vi "MALT132 output counter.vi"() -> ()   [LabVIEW 2018]
uses:
  <instrlib>/AltonTech MALT/Public/Types/MALT Family Codes.ctl
  <instrlib>/AltonTech MALT/AltonTech MALT200817.lvlib
panel:
  in  "Save":bool
  out "Kn Counter":u32
  in  "Address":i32=3 format="%02x"
  in  "Kn":i32=1
  in  "Kn":bool
  in  "stop":bool
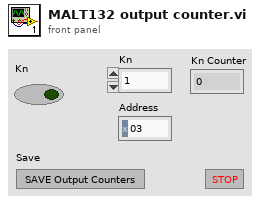
[diagram p1: front panel]
types:
  T1 = typedef "AltonTech MALT200817.lvlib/MALT Family Codes.ctl" = enum32{"-", "MALT40IO", "YAV904X8", "MALT132", "YAV91616", "MALT16PIN", "YAV90096", "YAV90HVT", "YAV90CLR", "YAV90128", "YAV90PNE", "MALTCON", "YAV91775", "YAV90XXX", "YAV90MMU", "H730050", "H710060", "H710061", "YAV90304", "MMI", "YAV90060", "MALT160T", "YAV90059", "Not Defined"}
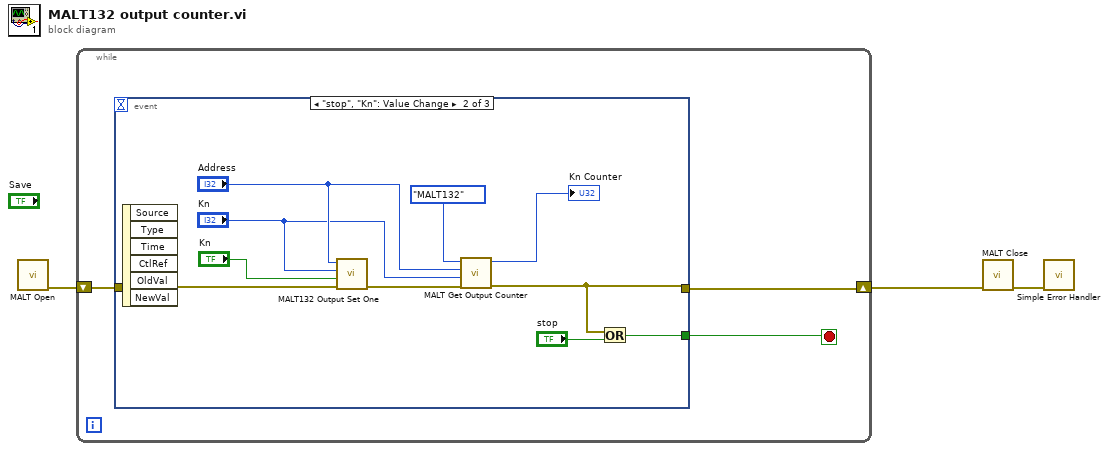
[diagram p0: block diagram]
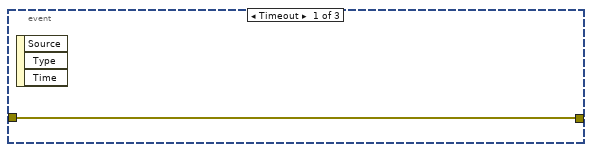
[diagram p2: hidden frame]
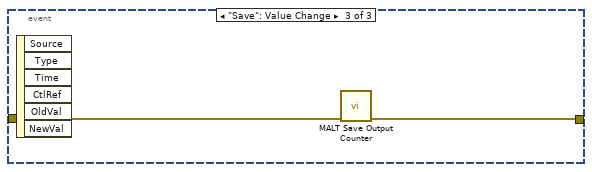
[diagram p3: hidden frame]
diagram:
  n1 = call <instrlib>:"MALT Open.vi"() -> ("error out"=w3:errorcluster)  [unwired: 10 in, 1 out]
  n2 = while {
    shift-right: [w5] -> w2
    shift-left: w3 -> [w6]
    stop <- w4 stop-if-true
    n3 = event shown="[1] \"stop\", \"Kn\": Value Change" {
      selector: _ -> [_ _ _]
      dyn-events: _ -> [_ _ _]
      timeout: _ -> [_ _ _]
      tunnel: w6 -> [w7 w16 w19]
      tunnel: [w7 w11 w18] -> w5
      tunnel: [_ w8 _] -> w4
      event Timeout {
        n4 = event-data() -> ()  [unwired: 1 in, 3 out]
      }
      event "stop", "Kn": Value Change {
        n5 = event-data() -> ()  [unwired: 1 in, 6 out]
        n6 = call <instrlib>:"MALT132 Output Set One.vi"("error in"=w16, "State"="Kn", "Kn"="Kn", "Address"="Address") -> ("error out"=w15:errorcluster)  [unwired: 7 in]
        n7 = call <instrlib>:"MALT Get Output Counter.vi"("error in"=w15, "Port"="Kn", "Address"="Address", "FamilyCode"=MALT_Family_Codes."MALT132") -> ("error out"=w11:errorcluster, "Value"=→"Kn Counter":u32)  [unwired: 6 in]
        n8 = Or(x=w11, y="stop") -> (x .or. y?=w8:bool)
      }
      event "Save": Value Change {
        n9 = event-data() -> ()  [unwired: 1 in, 6 out]
        n10 = call <instrlib>:"MALT Save Output Counter.vi"("error in"=w19) -> ("error out"=w18:errorcluster)  [unwired: 10 in]
      }
    }
  }
  n11 = call <instrlib>:"MALT Close.vi"("error in"=w2) -> ("error out"=w1:errorcluster)  [unwired: 10 in]
  n12 = call <vilib>:"Simple Error Handler.vi"("error in (no error)"=w1) -> ()  [unwired: 4 in, 5 out]
